vi "Set LED.vi"(0 "comm interface in":refnum<class "Pixy Com.lvclass">, 5 "color":cluster{"red":u8, "green":u8, "blue":u8}, 11 "error in":errorcluster) -> (4 "comm interface out":refnum<class "Pixy Com.lvclass">, 15 "error out":errorcluster)   [LabVIEW 2018, in "Pixy2.lvlib"]
uses:
  Pixy2.lvlib
  Interface/Pixy Com.lvclass
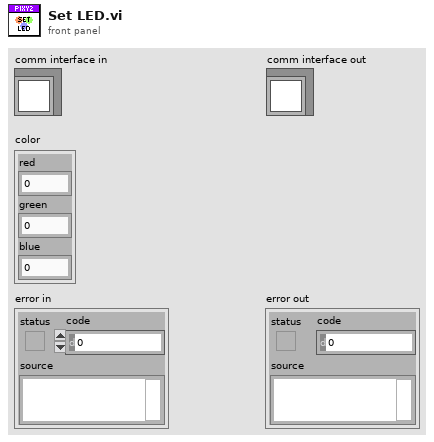
[diagram p1: front panel]
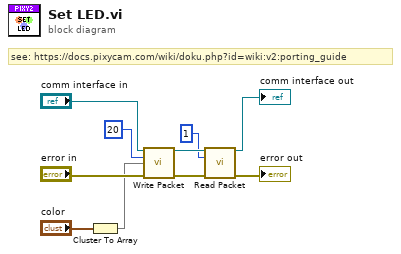
[diagram p0: block diagram]
diagram:
  # "see: https://docs.pixycam.com/wiki/doku.php?id=wiki:v2:porting_guide"
  n1 = Cluster To Array(cluster="color") -> (array=w7:u8[])
  n2 = call "Write Packet.vi"("comm interface in"="comm interface in", "type"=u8 20, "payload"=w7, "error in"="error in") -> ("comm interface out"=w5:refnum<class "Pixy Com.lvclass">, "error out"=w6:errorcluster)  [unwired: 10 in]
  n3 = call "Read Packet.vi"("comm interface in"=w5, "expected type"=u8 1, "error in"=w6) -> ("comm interface out"=→"comm interface out":refnum<class "Pixy Com.lvclass">, "error out"=→"error out":errorcluster)  [unwired: 9 in, 2 out]
